vi "ADI_IMU_ADIS16470_ScaleData.vi"(4 "Received Data":u8[](array[numeric])) -> (0 "Counter":u16, 1 "Data Array":dbl[](array[numeric]), 2 "Data Good?":bool)   [LabVIEW 2018, in "ADIS16470_IMU.lvlib"]
uses:
  ADIS16470_IMU.lvlib
panel:
  out "error out":errorcluster
  in  "error in (no error)":errorcluster
  out "Received Checksum":u16
  out "Calculated Checksum":u16
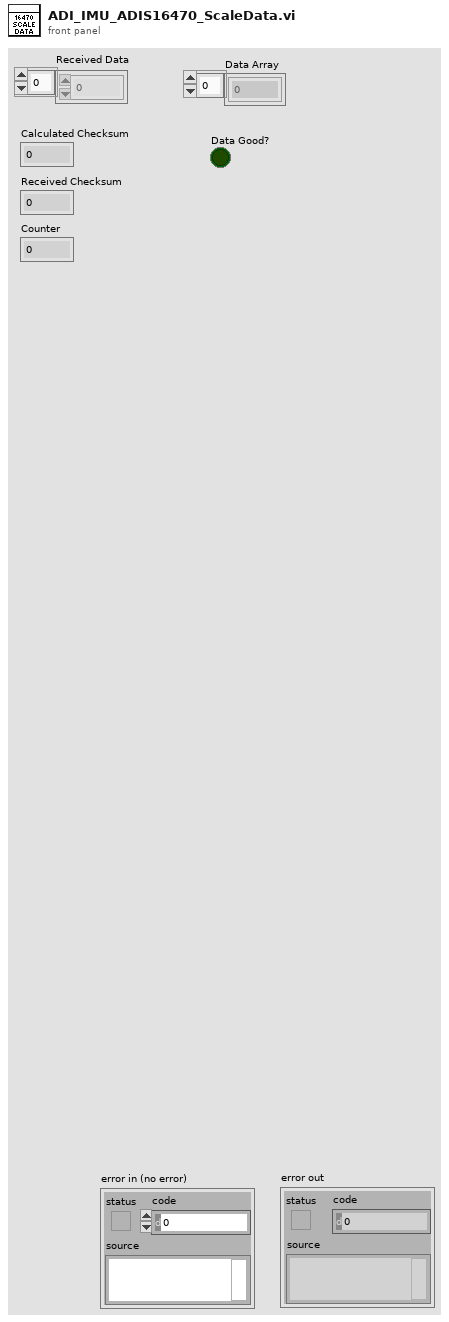
[diagram p1: front panel]
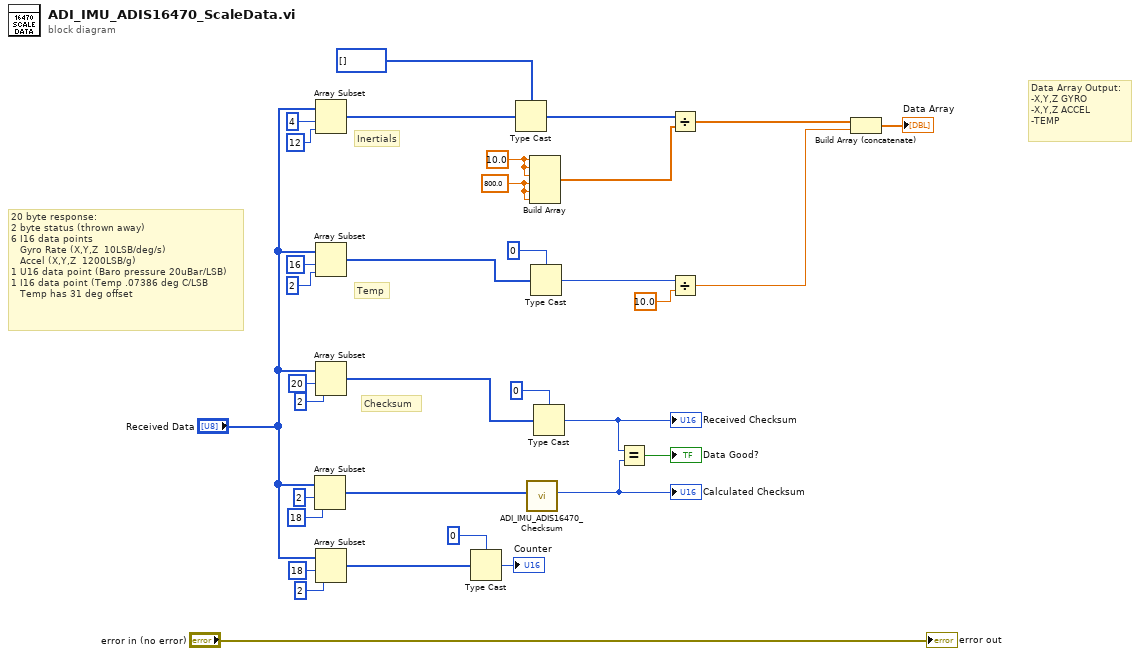
[diagram p0: block diagram]
diagram:
  w33 = 800.0
  w34 = 10.0 ("element")
  # "Checksum"
  # "Temp"
  # "Inertials"
  # "Data Array Output:\n-X,Y,Z GYRO\n-X,Y,Z ACCEL\n-TEMP"
  # "20 byte response:\n2 byte status (thrown away)\n6 I16 data points\n   Gyro Rate (X,Y,Z  10LSB/deg/s)\n   Accel (X,Y,Z  1200LSB/g)\n1 U16 data point (Baro pressure 20uBar/LSB)\n1 I16 data point (Temp .07386 deg C/LSB\n   Temp has 31 deg offset"
  n1 = Array Subset(array="Received Data", index=2, length=18) -> (w11:u8[])
  n2 = Array Subset(array="Received Data", index=4, length=12) -> (w21:u8[])
  n3 = Array Subset(array="Received Data", index=16, length=2) -> (w24:u8[])
  n4 = Array Subset(array="Received Data", index=20, length=2) -> (w15:u8[])
  n5 = Array Subset(array="Received Data", index=18, length=2) -> (w2:u8[])
  n6 = Type Cast(type=u16 0, x=w2) -> (*(type *) &x=→"Counter":u16)
  n7 = Type Cast(type=i16[] [], x=w21) -> (*(type *) &x=w20:i16[])
  n8 = call "ADI_IMU_ADIS16470_Checksum.vi"("Byte Array (MSB-First)"=w11) -> ("Checksum"=w9:u16)  [unwired: 10 in]
  "Calculated Checksum" <- w9
  n9 = Build Array(w34, w34, w34, w33, w33, w33) -> (w32:dbl[])
  n10 = Type Cast(type=i16 0, x=w24) -> (*(type *) &x=w22:i16)
  n11 = Type Cast(type=u16 0, x=w15) -> (*(type *) &x=w10:u16)
  "Received Checksum" <- w10
  n12 = Equal?(x=w10, y=w9) -> (x = y?=→"Data Good?":bool)
  n13 = Divide(x=w20, y=w32) -> (x/y=w30:dbl[])
  n14 = Divide(x=w22, y=10.0 ("element")) -> (x/y=w7:dbl)
  n15 = Build Array (concatenate)(w30, w7) -> (→"Data Array":dbl[])
  "error out" <- "error in (no error)"
